vi "Main Get Control Ref.vi"(8 "error in (no error)":errorcluster, 9 "Page Name":string, 10 "TabName":string="Settings", 11 "reference":refnum<vi>) -> (0 "error out":errorcluster, 2 "Output Array":string[](array[string]))   [LabVIEW 2022 SP3]
panel:
  in  "Filter":string
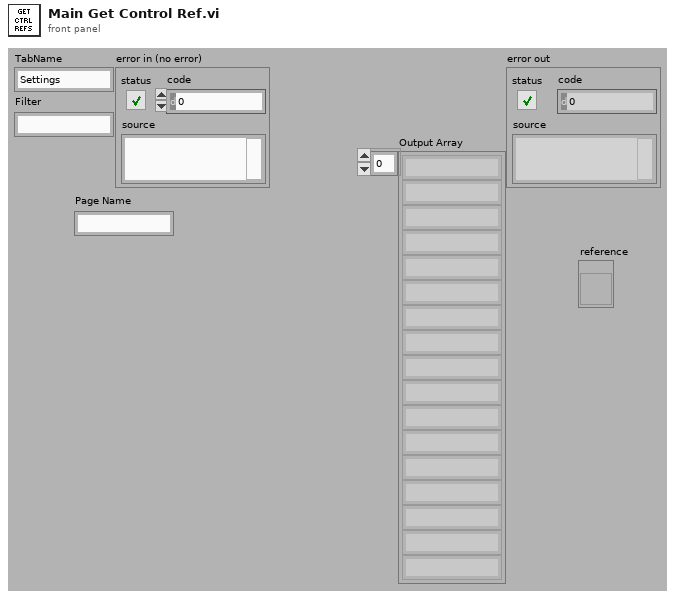
[diagram p1: front panel]
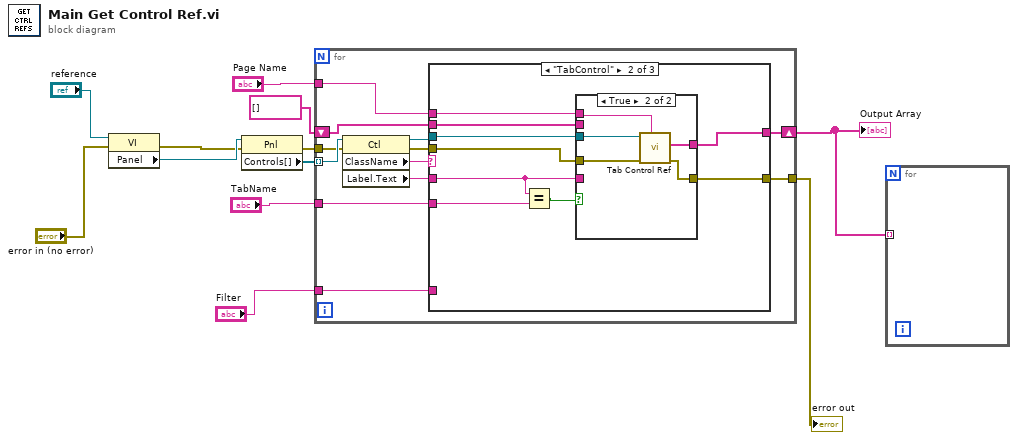
[diagram p0: block diagram]
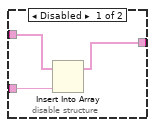
[diagram p3: hidden frame]
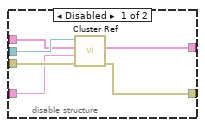
[diagram p6: hidden frame]
diagram:
  n1 = property class="VI"(reference="reference", error in="error in (no error)") -> (error out=w10:errorcluster, "Panel"=w12:refnum<vi>)  [unwired: 1 out]
  n2 = property class="Pnl"(reference=w12, error in=w10) -> (error out=w9:errorcluster, "Controls[]"=w11:refnum<vi>[])  [unwired: 1 out]
  n3 = for {
    tunnel: w11 -> [w24] mode=indexing
    tunnel: w9 -> [w23]
    shift-right: [w19] -> w1
    shift-left: string[] [] ("Array") -> [w18]
    tunnel: "Page Name" -> [w16]
    tunnel: "TabName" -> [w15]
    tunnel: [w14] -> w2
    tunnel: "Filter" -> [w13]
    n4 = property class="Ctl"(reference=w24, error in=w23) -> (reference out=w21:refnum<vi>, error out=w20:errorcluster, "ClassName"=w22:string, "Label.Text"=w17:string)
    n5 = case shown="\"TabControl\"" w22 {
      tunnel: w21 -> [_ w41 w54]
      tunnel: w20 -> [w25 w40 w53]
      tunnel: [w27 w38 w50] -> w19
      tunnel: w18 -> [w28 w39 w52]
      tunnel: w17 -> [w26 w37 w51]
      tunnel: w16 -> [_ w35 _]
      tunnel: w15 -> [_ w34 _]
      tunnel: [w25 w33 w49] -> w14
      tunnel: w13 -> [_ _ _]
      frame "", Default {
        n6 = disable-structure shown="Enabled" {
          disable-tunnel: w28 -> [w31 w32]
          disable-tunnel: [w30 w32] -> w27
          disable-tunnel: w26 -> [w29 _]
          frame Disabled {
            n7 = Insert Into Array(array=w31, new element=w29) -> (w30:string[])  [unwired: 1 in]
          }
          frame Enabled {
          }
        }
      }
      frame "TabControl" {
        n8 = Equal?(x=w37, y=w34) -> (x = y?=w36:bool)
        n9 = case shown="True" w36 {
          tunnel: w41 -> [_ w48]
          tunnel: w40 -> [w42 w47]
          tunnel: w39 -> [w43 _]
          tunnel: [w43 w46] -> w38
          tunnel: w37 -> [_ _]
          tunnel: w35 -> [_ w45]
          tunnel: [w42 w44] -> w33
          frame False {
          }
          frame True {
            n10 = call "Tab Control Ref.vi"("Page Label"=w45, "error in"=w47, "TabControl Reference"=w48) -> ("error out"=w44:errorcluster, "Array Out"=w46:string[])  [unwired: 6 in, 1 out]
          }
        }
      }
      frame "Cluster" {
        n11 = disable-structure shown="Enabled" {
          disable-tunnel: w54 -> [w60 _]
          disable-tunnel: w53 -> [w59 w61]
          disable-tunnel: w52 -> [w58 w62]
          disable-tunnel: w51 -> [w57 _]
          disable-tunnel: [w56 w62] -> w50
          disable-tunnel: [w55 w61] -> w49
          frame Disabled {
            n12 = call "Cluster Ref.vi"("error in"=w59, "Label Text"=w57, "Input Array"=w58, "Cluster Reference"=w60) -> ("error out"=w55:errorcluster, "Array Out"=w56:string[])  [unwired: 6 in]
          }
          frame Enabled {
          }
        }
      }
    }
  }
  "Output Array" <- w1
  "error out" <- w2
  n13 = for {
    tunnel: w1 -> [_] mode=indexing
  }
